vi "ZAlign_Delete_old_Decos.vi"(8 "error in (no error)":errorcluster, 10 "Decos[]":refnum<vi>[](array[refnum]), 11 "Panel in":refnum<vi>) -> (0 "error out":errorcluster, 3 "Panel out":refnum<vi> caption="Panel in")   [LabVIEW 2014, in "ZAlign.lvlib"]
doc: "ZAlign.lvlib:ZAlign_Delete_old_Decos.vi\n----------------------------------------------\nDelete old decorations\n\nInputs:\n---------------------\n- error in (no error) : Cluster; \n- Decos[] : 1DArrayOfRefnum; \n- Panel in : Refnum; \n\nOutputs:\n---------------------\n- error out : Cluster; \n\n----------------------------------------------\n16/03/2015\nZühlke Engineering AG\nCH-8952 Schlieren\nwww.zuehlke.com"
uses:
  ZAlign.lvlib
panel:
  # "Connector Pane"
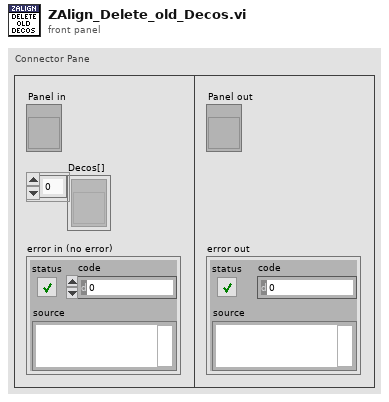
[diagram p1: front panel]
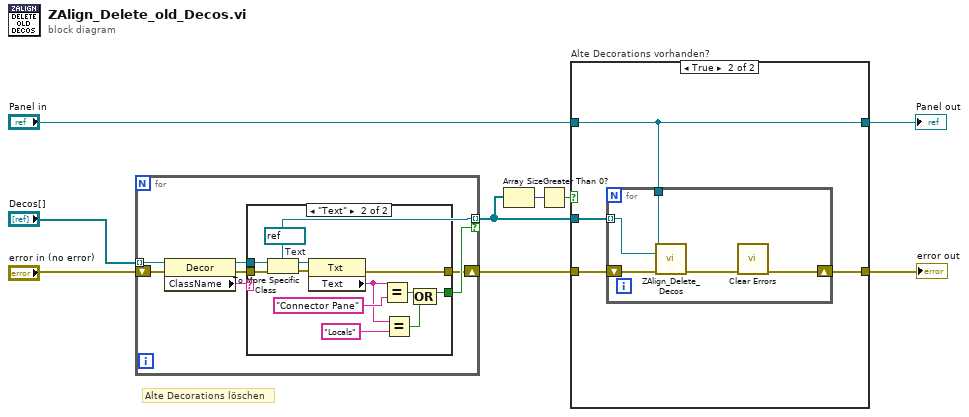
[diagram p0: block diagram]
diagram:
  # "Alte Decorations löschen"
  n1 = for {
    tunnel: "Decos[]" -> [w14] mode=indexing
    tunnel: [w12] -> w2 mode=indexing if=w16
    shift-right: [w15] -> w7
    shift-left: "error in (no error)" -> [w13]
    n2 = property class="Decor"(reference=w14, error in=w13) -> (reference out=w12:refnum<vi>, error out=w11:errorcluster, "ClassName"=w10:string)
    n3 = case shown="\"Text\"" w10 {
      tunnel: [_ w19] -> w16
      tunnel: [w17 w26] -> w15
      tunnel: w12 -> [_ w25]
      tunnel: w11 -> [w17 w24]
      frame Default {
      }
      frame "Text" {
        w29 = refnum<vi> refnum  # Text
        n4 = To More Specific Class(target class=w29, reference=w25, error in=w24) -> (specific class reference=w28:refnum<vi>, error out=w23:errorcluster)
        n5 = property class="Txt"(reference=w28, error in=w23) -> (error out=w26:errorcluster, "Text"=w22:string)  [unwired: 1 out]
        n6 = Equal?(x=w22, y="Connector Pane" ("Text")) -> (x = y?=w20:bool)
        n7 = Equal?(x=w22, y="Locals" ("Text")) -> (x = y?=w18:bool)
        n8 = Compound Arithmetic op=OR(w20, w18) -> (w19:bool)
      }
    }
  }
  n9 = Array Size(array=w2) -> (size(s)=w3:i32)
  n10 = Greater Than 0?(x=w3) -> (x > 0?=w4:bool)
  n11 = case "Alte Decorations vorhanden?" shown="True" w4 {
    tunnel: [w31 w35] -> w9
    tunnel: "Panel in" -> [w30 w33]
    tunnel: w7 -> [w31 w34]
    tunnel: w2 -> [_ w32]
    tunnel: [w30 w33] -> w1
    frame False {
    }
    frame True {
      n12 = for {
        tunnel: w33 -> [w39]
        shift-right: [w36] -> w35
        shift-left: w34 -> [w40]
        tunnel: w32 -> [w38] mode=indexing
        n13 = call "ZAlign_Delete_Decos.vi"("Panel in"=w39, "Decor Refnum"=w38, "error in (no error)"=w40) -> ("error out"=w37:errorcluster)  [unwired: 12 in]
        n14 = call <vilib>:"Clear Errors.vi"("error in (no error)"=w37) -> ("error out"=w36:errorcluster)  [unwired: 5 in, 1 out]
      }
    }
  }
  "error out" <- w9
  "Panel out" <- w1
